vi "Fire Laser.vi"(8 "error in (no error)":errorcluster, 10 "Laser Power":dbl, 11 "Recipe Process in":refnum<class "Recipe Process.lvclass">) -> (0 "error out":errorcluster, 3 "Recipe Process out":refnum<class "Recipe Process.lvclass">)   [LabVIEW 2022 SP3, in "Recipe Process.lvlib" / "Recipe Process.lvclass"]
uses:
  Recipe Process.lvclass
  Recipe Process.lvclass/Recipe Process.ctl
  Laser/Laser State Data/Laser State.ctl
  Laser/Laser State Data/Laser State Data.lvclass
  Laser/Laser Controller api/Laser API.lvclass
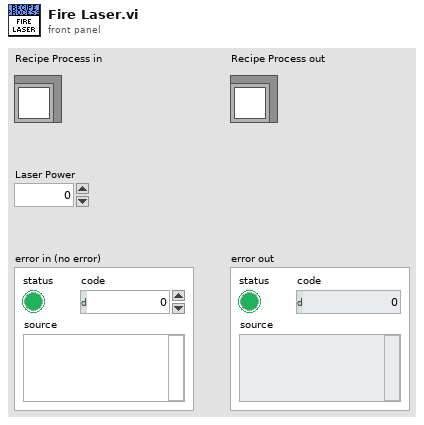
[diagram p1: front panel]
types:
  T1 = typedef "Laser State Data.lvclass/Laser State.ctl" = enum16{"Idle", "Warming", "Ready", "Firing"}
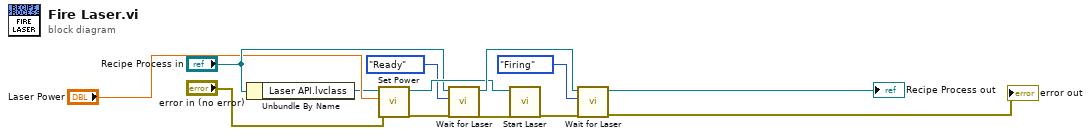
[diagram p0: block diagram]
diagram:
  n1 = Unbundle By Name("Recipe Process in") -> ("Laser API.lvclass"=w1:refnum<class "Laser API.lvclass">)
  n2 = call-dynamic "Set Power.vi"("error in (no error)"="error in (no error)", "Power"="Laser Power", "Laser API in"=w1) -> ("error out"=w5:errorcluster, "Laser API out"=w7:refnum<class "Laser API.lvclass">)  [unwired: 7 in]
  n3 = call "Wait for Laser.vi"("error in (no error)"=w5, "Desired State"=Laser_State."Ready" ("y"), "Recipe Process in"="Recipe Process in") -> ("error out"=w8:errorcluster, "Recipe Process out"=w9:refnum<class "Recipe Process.lvclass">)  [unwired: 7 in]
  n4 = call-dynamic "Start Laser.vi"("error in (no error)"=w8, "Laser API in"=w7) -> ("error out"=w11:errorcluster)  [unwired: 8 in, 1 out]
  n5 = call "Wait for Laser.vi"("error in (no error)"=w11, "Desired State"=Laser_State."Firing", "Recipe Process in"=w9) -> ("error out"=→"error out":errorcluster, "Recipe Process out"=→"Recipe Process out":refnum<class "Recipe Process.lvclass">)  [unwired: 7 in]
